vi "Test Complete Coverage.vi"(8 "error in (no error)":errorcluster, 11 "Test Case In":refnum<class "Coverage Test.lvclass">) -> (0 "error out":errorcluster, 3 "Test Case Out":refnum<class "Coverage Test.lvclass">)   [LabVIEW 2020, in "LUnit Tests.lvlib" / "Coverage Test.lvclass"]
uses:
  Coverage Test.lvclass
  C:/Program Files (x86)/National Instruments/LabVIEW 2020/vi.lib/Astemes/LUnit/Test Case.lvclass
  source/Framework/Coverage Analyzer/Coverage Analyzer.lvclass
  <vilib>/Astemes/LUnit/Test Case.lvclass/Test Case.ctl
  <vilib>/Astemes/LUnit/LUnit Assertion Result.lvclass/LUnit Assertion Result.ctl
  <vilib>/Astemes/LUnit/LUnit Test Case Result.lvclass/LUnit Test Case Result.ctl
  <vilib>/Astemes/LUnit/LUnit Method Result.lvclass/LUnit Method Result.ctl
  01074fa8-ee8a-411d-bc8b-fc92c4f90959.vi
  <vilib>/Astemes/LUnit/Set Assertion Type.vi
  <vilib>/Astemes/LUnit/Palette/Pass.vi
  <vilib>/Astemes/LUnit/Palette/Fail.vi
  <vilib>/Astemes/LUnit/Compare Variants.vi
  <vilib>/Astemes/LUnit/Describe Comparison.vi
  <vilib>/Astemes/LUnit/LUnit Write Assertion Type.vi
  <vilib>/Astemes/LUnit/Add test result.vi
  <vilib>/Astemes/LUnit/LUnit Write Passed.vi
  <vilib>/Astemes/LUnit/LUnit Write Message.vi
  <vilib>/Astemes/LUnit/LUnit Write Description.vi
  <vilib>/Astemes/LUnit/Variant to string.vi
  <vilib>/Astemes/LUnit/LUnit Record Assertion Result.vi
  <vilib>/Astemes/LUnit/LUnit Aggregate Assertion Results.vi
  <vilib>/Astemes/LUnit/Assertion Result/LUnit Read Status.vi
  <vilib>/Astemes/LUnit/LUnit Read Message.vi
  <vilib>/Astemes/LUnit/LUnit Read Description.vi
  <vilib>/Astemes/LUnit/Method Result/LUnit Merge Status.vi
  <vilib>/Astemes/LUnit/LUnit Concatenate result strings.vi
  <vilib>/Utility/Data Type/Get Type Information.vi
  <vilib>/Utility/LVClass/Get LV Class Name.vi
  <vilib>/Astemes/LUnit/LUnit Assertion Result.lvclass
  Coverage Test.lvclass/Coverage Test.ctl
  <vilib>/Astemes/LUnit/Test Case.lvclass
  C:/Git/astemes-lunit/tests/Coverage Test/Coverage Test.lvclass
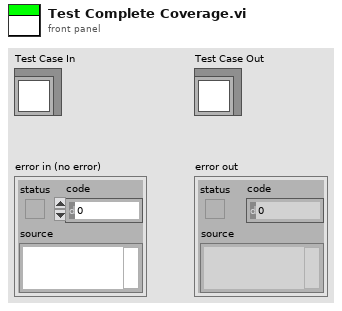
[diagram p1: front panel]
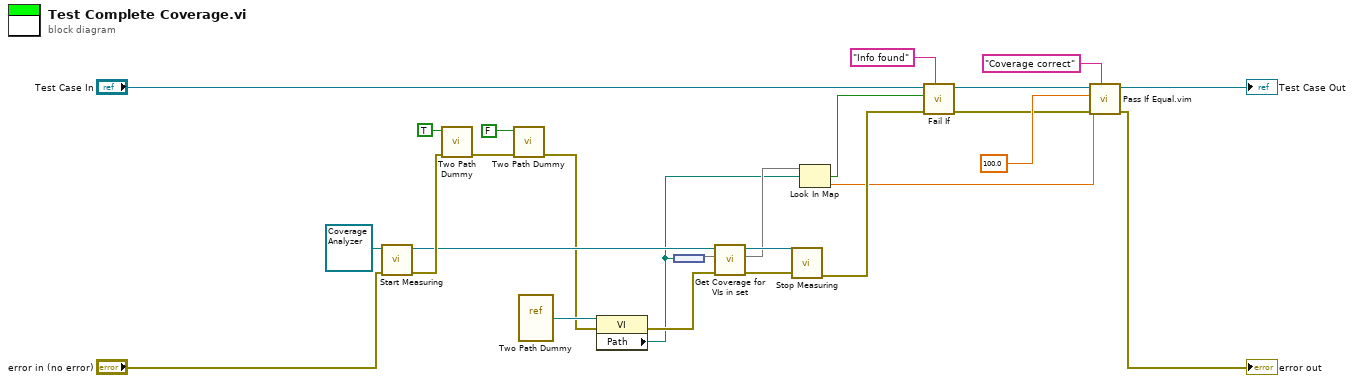
[diagram p0: block diagram]
diagram:
  n1 = call "Start Measuring.vi"("error in (no error)"="error in (no error)", "Coverage Analyzer in"=refnum<class "Coverage Analyzer.lvclass"> refnum) -> ("error out"=w17:errorcluster, "Coverage Analyzer out"=w16:refnum<class "Coverage Analyzer.lvclass">)  [unwired: 8 in]
  n2 = call "Two Path Dummy.vi"("error in (no error)"=w17, "Boolean"=TRUE) -> ("error out"=w21:errorcluster)  [unwired: 9 in]
  n3 = call "Two Path Dummy.vi"("error in (no error)"=w21, "Boolean"=FALSE) -> ("error out"=w6:errorcluster)  [unwired: 9 in]
  n4 = vi-ref "Two Path Dummy.vi"() -> (w24:refnum<vi>)
  n5 = property class="VI"(reference=w24, error in=w6) -> (error out=w7:errorcluster, "Path"=w1:path)  [unwired: 1 out]
  n6 = node(w1) -> (w2:set{path})
  n7 = call "Get Coverage for VIs in set.vi"("error in (no error)"=w7, "VIs"=w2, "Coverage Analyzer in"=w16) -> ("error out"=w14:errorcluster, "Code Coverage"=w4:map{path, dbl}, "Coverage Analyzer out"=w15:refnum<class "Coverage Analyzer.lvclass">)  [unwired: 6 in]
  n8 = call "Stop Measuring.vi"("error in (no error)"=w14, "Coverage Analyzer in"=w15) -> ("error out"=w10:errorcluster)  [unwired: 8 in, 1 out]
  n9 = Look In Map(map=w4, key=w1) -> (key not found?=w3:bool, value=w5:dbl)  [unwired: 1 in]
  n10 = call <vilib>:"Fail If.vi"("Description"="Info found", "error in (no error)"=w10, "Fail?"=w3, "LUnit Test Case In"="Test Case In") -> ("error out"=w13:errorcluster, "LUnit Test Case Out"=w11:refnum<class "Coverage Test.lvclass">)  [unwired: 6 in]
  n11 = call "Pass If Equal.vim"("Description"="Coverage correct", "error in (no error)"=w13, "Actual"=w5, "Expected"=100.0 ("Coverage Percentage"), "LUnit Test Case In"=w11) -> ("error out"=→"error out":errorcluster, "LUnit Test Case Out"=→"Test Case Out":refnum<class "Coverage Test.lvclass">)  [unwired: 5 in]
